vi "Calc UV Start Deltas.vi"(7 "Texture Dimensions":T3, 10 "UVs":cluster{"Top":T2, "Middle":T2, "Bottom":T2} {"Bottom"."v" min=0 max=1 step=0.1; "Bottom"."u" min=0 max=1 step=0.1; "Middle"."v" min=0 max=1 step=0.1; "Middle"."u" min=0 max=1 step=0.1; "Top"."v" min=0 max=1 step=0.1; "Top"."u" min=0 max=1 step=0.1}, 11 "Vertices":cluster{"Top":T1, "Middle":T1, "Bottom":T1}) -> (3 "Start Deltas (Pixels)":T2 {"v" min=0 max=1 step=0.1; "u" min=0 max=1 step=0.1})   [LabVIEW 2022 SP3]
uses:
  Raster.lvlib
  UV.ctl
  Point 2D.ctl
  Rectangle Dimensions.ctl
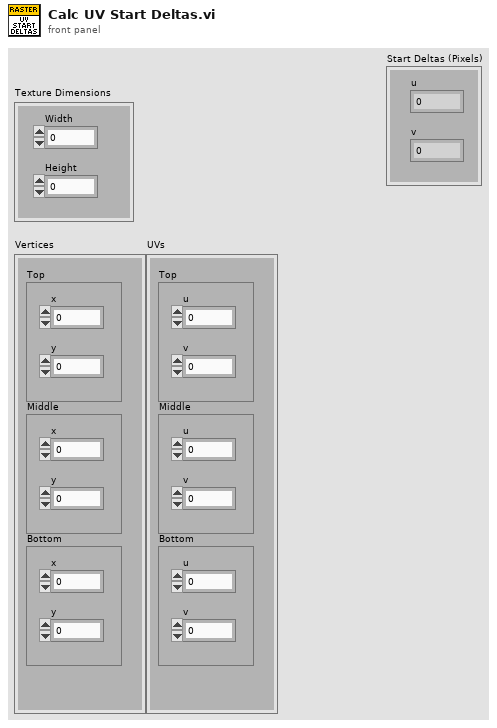
[diagram p1: front panel]
types:
  T1 = typedef "Raster.lvlib/Point 2D.ctl" = cluster{"x":i32, "y":i32}
  T2 = typedef "Raster.lvlib/UV.ctl" = cluster{"u":sgl, "v":sgl}
  T3 = typedef "Raster.lvlib/Rectangle Dimensions.ctl" = cluster{"Width":u32, "Height":u32}
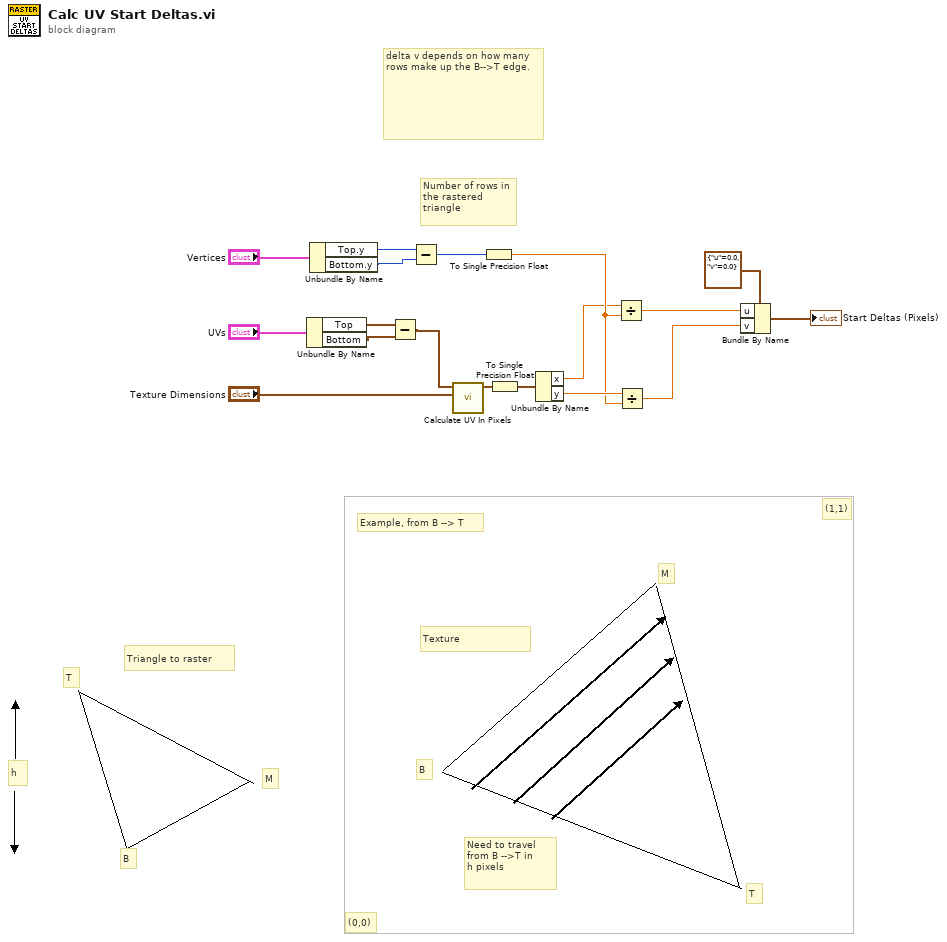
[diagram p0: block diagram]
diagram:
  # "Example, from B --> T"
  # "(0,0)"
  # "(1,1)"
  # "h"
  # "Texture"
  # "Triangle to raster"
  # "M"
  # "T"
  # "B"
  # "Need to travel from B -->T in \nh pixels"
  # "Number of rows in the rastered triangle"
  # "delta v depends on how many rows make up the B-->T edge."
  # "T"
  # "M"
  # "B"
  n1 = Unbundle By Name("UVs") -> ("Top"=w11:T2, "Bottom"=w10:T2)
  n2 = Unbundle By Name("Vertices") -> ("Top.y"=w13:i32, "Bottom.y"=w12:i32)
  n3 = Subtract(x=w11, y=w10) -> (x-y=w9:T2)
  n4 = Subtract(x=w13, y=w12) -> (x-y=w8:i32)
  n5 = call "Calculate UV In Pixels.vi"(10:"Texture Dimensions", "UV"=w9) -> ("Pixels"=w7:T1)  [unwired: 9 in]
  n6 = To Single Precision Float(number=w8) -> (single precision float=w4:sgl)
  n7 = To Single Precision Float(number=w7) -> (single precision float=w6:cluster{"x":sgl, "y":sgl})
  n8 = Unbundle By Name(w6) -> ("x"=w3:sgl, "y"=w5:sgl)
  n9 = Divide(x=w3, y=w4) -> (x/y=w2:sgl)
  n10 = Divide(x=w5, y=w4) -> (x/y=w1:sgl)
  n11 = Bundle By Name(cluster=T2 {"u"=0.0, "v"=0.0} ("Start Deltas"), "u"=w2, "v"=w1) -> (→"Start Deltas (Pixels)":T2)
